vi "ConversaoU32 para matriz 16.vi"(1 "Número [U32]":i32) -> (0 "Array 2*[U16]":u16[](array[numeric]))   [LabVIEW 2019]
panel:
  out "Boolean array 2":bool[](array[boolean])
  out "Boolean array":bool[](array[boolean])
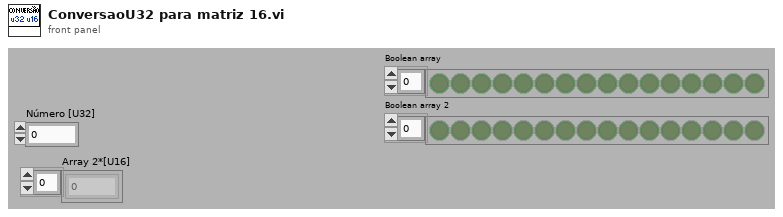
[diagram p1: front panel]
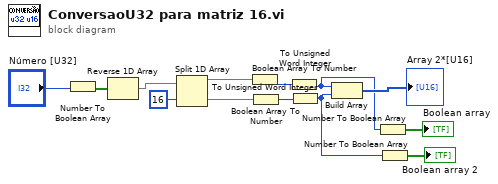
[diagram p0: block diagram]
diagram:
  n1 = Number To Boolean Array(number="Número [U32]") -> (Boolean array=w4:bool[])
  n2 = Reverse 1D Array(array=w4) -> (reversed array=w3:bool[])
  n3 = Split 1D Array(array=w3, index=16) -> (first subarray=w12:bool[], second subarray=w13:bool[])
  n4 = Boolean Array To Number(Boolean array=w12) -> (number=w2:u32)
  n5 = Boolean Array To Number(Boolean array=w13) -> (number=w1:u32)
  n6 = To Unsigned Word Integer(number=w2) -> (unsigned 16bit integer=w8:u16)
  n7 = To Unsigned Word Integer(number=w1) -> (unsigned 16bit integer=w7:u16)
  n8 = Build Array(w8, w7) -> (→"Array 2*[U16]":u16[])
  n9 = Number To Boolean Array(number=w8) -> (Boolean array=→"Boolean array":bool[])
  n10 = Number To Boolean Array(number=w7) -> (Boolean array=→"Boolean array 2":bool[])
